vi "Close Connection.vi"(8 "error in":errorcluster, 11 "uService Template in":refnum<class "TCP Listener.lvclass">) -> (0 "error out":errorcluster, 3 "uService Template out":refnum<class "TCP Listener.lvclass">)   [LabVIEW 2020, in "TALOS.lvlib" / "TCP Listener.lvlib" / "TCP Listener.lvclass"]
uses:
  TCP Listener.lvclass
  TCP Listener.lvclass/TCP Listener.ctl
  TALOS.lvlib
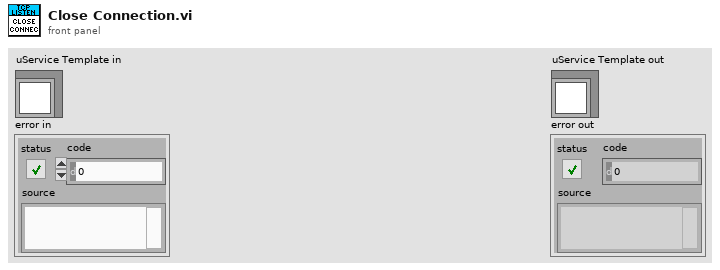
[diagram p1: front panel]
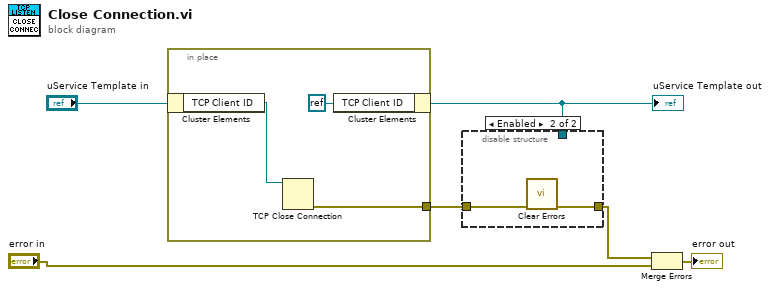
[diagram p0: block diagram]
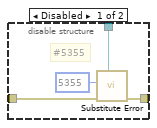
[diagram p2: hidden frame]
diagram:
  n1 = in-place {
    in-place-border: [w9] -> w4
    n2 = in-place-cluster #1("uService Template in") -> ("TCP Client ID"=w8:refnum<k5>)
    n3 = TCP Close Connection(connection ID=w8) -> (error out=w9:errorcluster)  [unwired: 2 in, 1 out]
    n4 = in-place-cluster #1("TCP Client ID"=refnum<k0> refnum) -> (w1:refnum<class "TCP Listener.lvclass">)
  }
  "uService Template out" <- w1
  n5 = disable-structure shown="Enabled" {
    disable-tunnel: w4 -> [w13 w15]
    disable-tunnel: [w12 w14] -> w3
    disable-tunnel: w1 -> [w11 _]
    frame Disabled {
      # "#5355"
      n6 = call "Substitute Error.vi"("LabVIEW Object"=w11, "error in (no error)"=w13, "Error Code"=5355) -> ("error out"=w12:errorcluster)  [unwired: 8 in]
    }
    frame Enabled {
      n7 = call <vilib>:"Clear Errors.vi"("error in (no error)"=w15) -> ("error out"=w14:errorcluster)  [unwired: 5 in, 1 out]
    }
  }
  n8 = Merge Errors(w3, "error in") -> (→"error out":errorcluster)
